vi "获得消息.vi"(11 "messages":T1[](array[typedef])) -> (3 "连接的字符串":string)   [LabVIEW 2012]
uses:
  <vilib>/LabVIEW Targets/Embedded/WSN/Host API/WSN Message.ctl
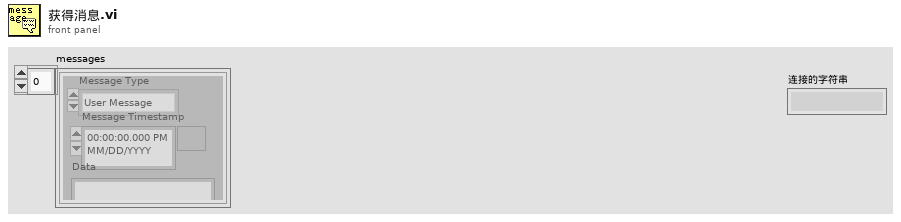
[diagram p1: front panel]
types:
  T1 = typedef "WSN Message.ctl" = cluster{"Message Type":enum16{"User Message", "Debug Message"}, "Message Timestamp":timestamp, "Data":string}
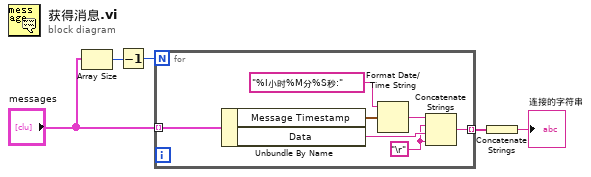
[diagram p0: block diagram]
diagram:
  n1 = Array Size(array="messages") -> (size(s)=w4:i32)
  n2 = Decrement(x=w4) -> (x-1=w3:i32)
  n3 = for {
    N: w3 -> [_]
    tunnel: "messages" -> [w8] mode=indexing
    tunnel: [w6] -> w2 mode=indexing
    w7 = "\r"
    n4 = Unbundle By Name(w8) -> ("Message Timestamp"=w10:timestamp, "Data"=w12:string)
    n5 = Format Date/Time String(time format string (%c)="%I小时%M分%S秒:" ("时间格式字符串(%c)"), seconds (now)=w10) -> (date/time string=w11:string)  [unwired: 1 in]
    n6 = Concatenate Strings(w11, w7, w12, w7) -> (w6:string)
  }
  n7 = Concatenate Strings(w2) -> (→"连接的字符串":string)
